vi "测试模块.vi"() -> ()   [LabVIEW 2015]
uses:
  kormeedb_api/my_config/global_config.vi
panel:
  out "默认上传数据输出":string[](array[string])
  out "配置信息输出":T1
  out "上传反馈结果":string
  out "数据库连接状态：":bool
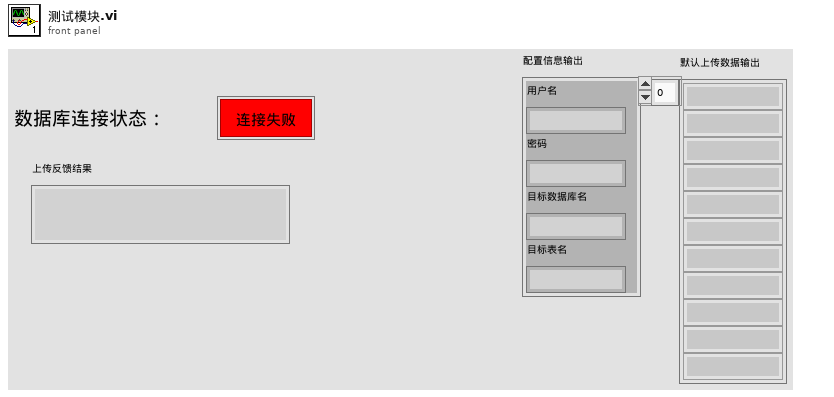
[diagram p1: front panel]
types:
  T1 = cluster{"用户名":string, "密码":string, "目标数据库名":string, "目标表名":string}
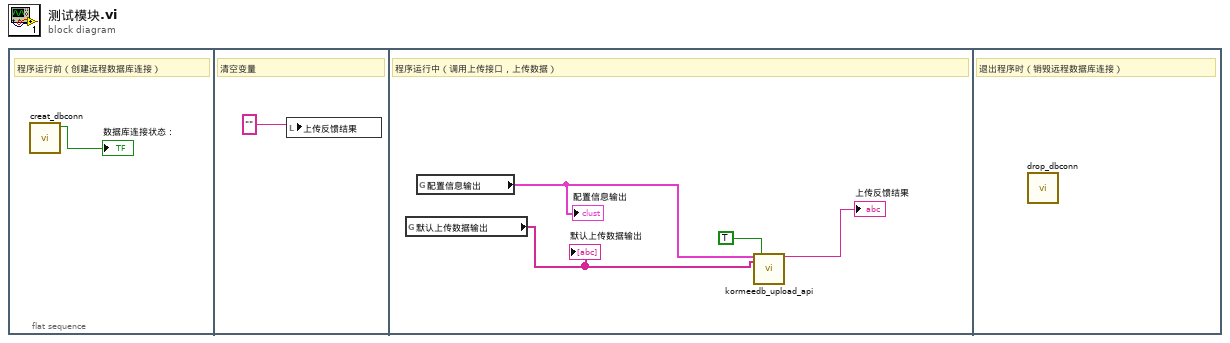
[diagram p0: block diagram]
diagram:
  n1 = flat-sequence {
    frame #0 {
      # "程序运行前（创建远程数据库连接）"
      n2 = call "creat_dbconn.vi"() -> ("连接结果"=→"数据库连接状态：":bool)  [unwired: 9 in, 2 out]
    }
    frame #1 {
      # "清空变量"
      n3 = local write "上传反馈结果"("") -> ()
    }
    frame #2 {
      # "程序运行中（调用上传接口，上传数据）"
      n4 = global read "global_config.vi" "默认上传数据输出"() -> (w4:string[])
      "默认上传数据输出" <- w4
      n5 = global read "global_config.vi" "配置信息输出"() -> (w3:T1)
      "配置信息输出" <- w3
      n6 = call "kormeedb_upload_api.vi"("上传信息输入"=w3, "要上传的数据"=w4, "数据存在则替换?"=TRUE) -> ("操作结果"=→"上传反馈结果":string)  [unwired: 14 in, 2 out]
    }
    frame #3 {
      # "退出程序时（销毁远程数据库连接）"
      n7 = call "drop_dbconn.vi"() -> ()  [unwired: 10 in, 2 out]
    }
  }
